vi "GPIB_Serial_Number.vi"(6 "Simulation data":string, 8 "Error In":errorcluster, 10 "Simulation":bool, 11 "GPIB Address":string="1") -> (0 "Error Out":errorcluster, 2 "Model":string, 3 "Serial Number":string)   [LabVIEW 2010]
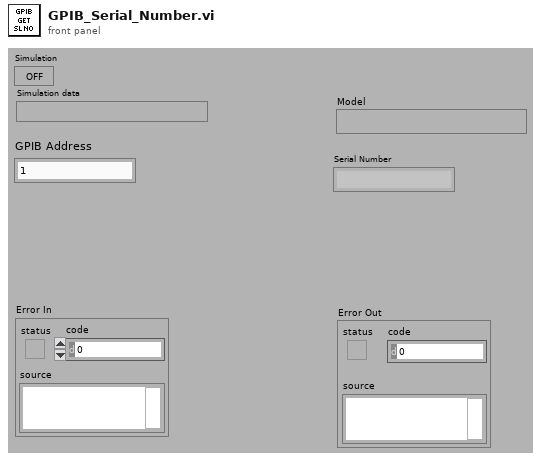
[diagram p1: front panel]
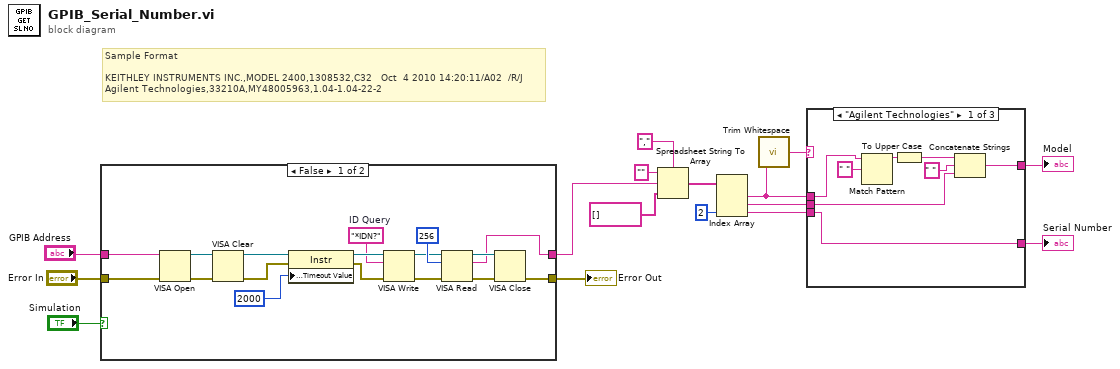
[diagram p0: block diagram]
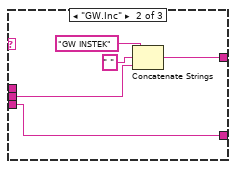
[diagram p2: hidden frame]
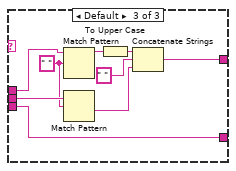
[diagram p3: hidden frame]
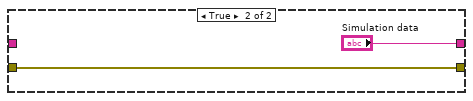
[diagram p4: hidden frame]
diagram:
  # "Sample Format\n\nKEITHLEY INSTRUMENTS INC.,MODEL 2400,1308532,C32   Oct  4 2010 14:20:11/A02  /R/J\nAgilent Technologies,33210A,MY48005963,1.04-1.04-22-2"
  n1 = case shown="False" "Simulation" {
    tunnel: "GPIB Address" -> [w20 _]
    tunnel: [w18 w35] -> w1
    tunnel: "Error In" -> [w19 w35]
    tunnel: [w17 "Simulation data"] -> w7
    frame False {
      w24 = "*IDN?"  # ID Query
      n2 = VISA Open(error in (no error)=w19, VISA resource name=w20) -> (VISA resource name=w29:refnum<visa-resource-name>, error out=w30:errorcluster)  [unwired: 3 in]
      n3 = VISA Clear(VISA resource name=w29, error in (no error)=w30) -> (VISA resource name out=w26:refnum<visa-resource-name>, error out=w27:errorcluster)
      n4 = property class="Instr"(reference=w26, error in=w27, "General Settings:Timeout Value"=u32 2000) -> (reference out=w28:refnum<visa-resource-name>, error out=w31:errorcluster)
      n5 = VISA Write(VISA resource name=w28, write buffer=w24, error in (no error)=w31) -> (VISA resource name out=w21:refnum<visa-resource-name>, error out=w22:errorcluster)  [unwired: 1 out]
      n6 = VISA Read(VISA resource name=w21, byte count=u32 256, error in (no error)=w22) -> (VISA resource name out=w32:refnum<visa-resource-name>, read buffer=w17:string, error out=w33:errorcluster)  [unwired: 1 out]
      n7 = VISA Close(VISA resource name=w32, error in (no error)=w33) -> (error out=w18:errorcluster)
    }
    frame True {
    }
  }
  "Error Out" <- w1
  n8 = Spreadsheet String To Array(delimiter (Tab)=",", format string="", spreadsheet string=w7, array type (2D Dbl)=string[] []) -> (array=w11:string[])
  n9 = Index Array(array=w11, index #3=2 ("index")) -> (element #1=w5:string, element #2=w8:string, element #3=w9:string)  [unwired: 2 in]
  n10 = call <vilib>:"Trim Whitespace.vi"("string"=w5) -> ("trimmed string"=w2:string)  [unwired: 1 in]
  n11 = case shown="\"Agilent Technologies\"" w2 {
    tunnel: w9 -> [w39 w47 w51]
    tunnel: w5 -> [w43 _ w57]
    tunnel: w8 -> [w37 w45 w56]
    tunnel: [w39 w47 w51] -> w4
    tunnel: [w38 w46 w50] -> w3
    frame "Agilent Technologies" {
      n12 = Match Pattern(string=w43, regular expression=" ") -> (before substring=w42:string)  [unwired: 1 in, 3 out]
      n13 = To Upper Case(1:w42) -> (0:w36:string)
      n14 = Concatenate Strings(w36, " " ("regular expression"), w37) -> (w38:string)
    }
    frame "GW.Inc" {
      n15 = Concatenate Strings("GW INSTEK" ("string"), " " ("regular expression"), w45) -> (w46:string)
    }
    frame Default {
      w54 = " " ("regular expression")
      n16 = Match Pattern(string=w57, regular expression=w54) -> (before substring=w55:string)  [unwired: 1 in, 3 out]
      n17 = Match Pattern(string=w56, regular expression=w54) -> (after substring=w52:string)  [unwired: 1 in, 3 out]
      n18 = To Upper Case(1:w55) -> (0:w49:string)
      n19 = Concatenate Strings(w49, " " ("regular expression"), w52) -> (w50:string)
    }
  }
  "Serial Number" <- w4
  "Model" <- w3
